vi "Filter Log Packet.vi"(10 "Log Packet":T1, 11 "Compound Filter in":refnum<class "Event Source Filter.lvclass">) -> (2 "Log?":bool, 3 "Compound Filter out":refnum<class "Event Source Filter.lvclass">)   [LabVIEW 2019, in "Event Source Filter.lvclass"]
uses:
  <vilib>/gpm_packages/@cs/event-logger/Source/Filters/Event Source Filter/Event Source Filter.lvclass
  <vilib>/gpm_packages/@cs/event-logger/Source/Composed Log/Types/Log Packet.ctl
  <vilib>/gpm_packages/@cs/event-logger/Source/Composed Log/Types/Log Level.ctl
  <vilib>/gpm_packages/@cs/event-logger/Source/Filters/Event Source Filter/Event Source Filter.lvclass/Event Source Filter.ctl
  <vilib>/gpm_packages/@cs/event-logger/Source/Composed Log/Composed Log.lvlib
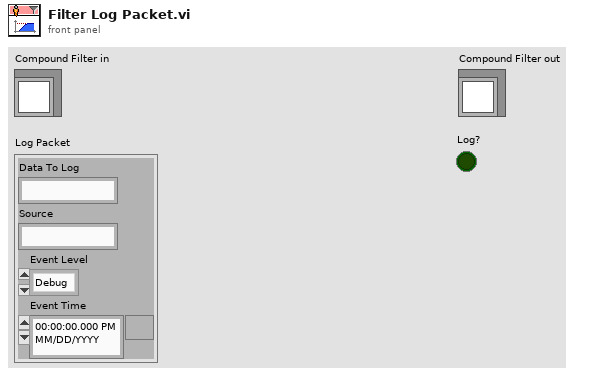
[diagram p1: front panel]
types:
  T1 = typedef "Composed Log.lvlib/Log Packet.ctl" = cluster{"Data To Log":string, "Source":string, "Event Level":T2, "Event Time":timestamp}
  T2 = typedef "Composed Log.lvlib/Log Level.ctl" = enum16{"Debug", "Info", "Warning", "Error", "Critical"}
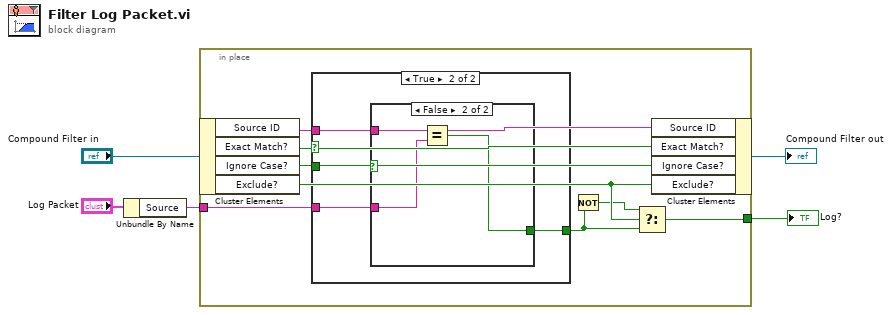
[diagram p0: block diagram]
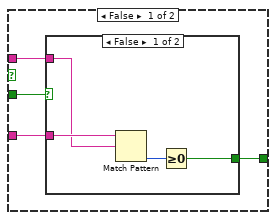
[diagram p2: hidden frame]
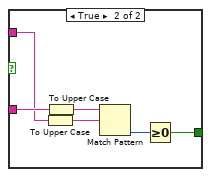
[diagram p3: hidden frame]
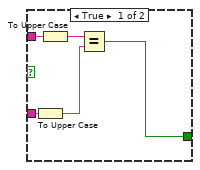
[diagram p4: hidden frame]
diagram:
  n1 = Unbundle By Name("Log Packet") -> ("Source"=w1:string)
  n2 = in-place {
    in-place-border: [w6] -> w5
    in-place-border: w1 -> [w11]
    n3 = in-place-cluster #1("Compound Filter in") -> ("Source ID"=w12:string, "Exact Match?"=w10:bool, "Ignore Case?"=w13:bool, "Exclude?"=w9:bool)
    n4 = case shown="True" w10 {
      tunnel: [w15 w29] -> w7
      tunnel: w13 -> [w14 w28]
      tunnel: w12 -> [w16 w31]
      tunnel: w11 -> [w17 w30]
      frame False {
        n5 = case shown="False" w14 {
          tunnel: w17 -> [w21 w27]
          tunnel: w16 -> [w20 w26]
          tunnel: [w18 w24] -> w15
          frame False {
            n6 = Match Pattern(string=w21, regular expression=w20) -> (offset past match=w19:i32)  [unwired: 1 in, 3 out]
            n7 = Greater Or Equal To 0?(x=w19) -> (x >= 0?=w18:bool)
          }
          frame True {
            n8 = To Upper Case(1:w26) -> (0:w22:string)
            n9 = To Upper Case(1:w27) -> (0:w23:string)
            n10 = Match Pattern(string=w23, regular expression=w22) -> (offset past match=w25:i32)  [unwired: 1 in, 3 out]
            n11 = Greater Or Equal To 0?(x=w25) -> (x >= 0?=w24:bool)
          }
        }
      }
      frame True {
        n12 = case shown="False" w28 {
          tunnel: w31 -> [w36 w37]
          tunnel: w30 -> [w35 w38]
          tunnel: [w34 w39] -> w29
          frame True {
            n13 = To Upper Case(1:w35) -> (0:w32:string)
            n14 = To Upper Case(1:w36) -> (0:w33:string)
            n15 = Equal?(x=w33, y=w32) -> (x = y?=w34:bool)
          }
          frame False {
            n16 = Equal?(x=w37, y=w38) -> (x = y?=w39:bool)
          }
        }
      }
    }
    n17 = Not(x=w7) -> (.not. x?=w8:bool)
    n18 = Select(t=w8, s=w9, f=w7) -> (s? t:f=w6:bool)
    n19 = in-place-cluster #1("Source ID"=w12, "Exact Match?"=w10, "Ignore Case?"=w13, "Exclude?"=w9) -> (→"Compound Filter out":refnum<class "Event Source Filter.lvclass">)
  }
  "Log?" <- w5
